vi "Periodic Tasks.vi"(8 "error in":errorcluster) -> ()   [LabVIEW 2020]
doc: "This VI runs in parallel to other tasks. It can contain as many user-defined periodic loops as you need. These can carry out PID or other sorts of timed response."
uses:
  <vilib>/Rock Robotics/WPI/ThirdParty/JAS_Junk/TrajLib/TypeDef/POSE2D.ctl
  <vilib>/Rock Robotics/WPI/ThirdParty/JAS_Junk/TrajLib/TypeDef/TRANSLATION2D.ctl
  <vilib>/Rock Robotics/WPI/ThirdParty/JAS_Junk/TrajLib/TypeDef/ROTATION2D.ctl
  <vilib>/Rock Robotics/WPI/ThirdParty/JAS_Junk/TrajLib/TypeDef/SWERVE_DRIVE_ODOMETRY.ctl
  <vilib>/Rock Robotics/WPI/ThirdParty/JAS_Junk/TrajLib/TypeDef/SWERVE_DRIVE_MODULE_POSITION.ctl
  <vilib>/Rock Robotics/WPI/ThirdParty/Phoenix-LabVIEW/Motor Controller/Controls/CTRE_Phoenix_MotorControl_ControlMode.ctl
  Robot Global Data.vi
  <vilib>/Rock Robotics/WPI/ThirdParty/Phoenix-LabVIEW/CANCoder/Get/CTRE_Phoenix_CANcoder_GetSensorData.vi
  <vilib>/Rock Robotics/WPI/ThirdParty/Phoenix-LabVIEW/Pigeon IMU/CTRE_PigeonIMU_GetAccumGyro.vi
  <vilib>/Rock Robotics/WPI/ThirdParty/Phoenix-LabVIEW/Motor Controller/Get/CTRE_Phoenix_MotorController_IntegratedSensorData_TalonFX.vi
  <vilib>/Rock Robotics/WPI/ThirdParty/JAS_Junk/TrajLib/Trajectory_Library.lvlib
panel:
  out "out SWERVE_DRIVE_ODOMETRY":T1={"POSE"={"TRANSLATION"={"X"=0.0, "Y"=0.0}, "ROTATION"={"VALUE"=0.0, "COS"=1.0, "SIN"=0.0}}, "GyroOffset"={"VALUE"=0.0, "COS"=1.0, "SIN"=0.0}, "PreviousAngle"={"VALUE"=0.0, "COS"=1.0, "SIN"=0.0}, "PrevModulePositions"=[], "NumModules"=0} {"PrevModulePositions"."Angle"."SIN" format="%13.4f"; "PrevModulePositions"."Angle"."COS" format="%13.4f"; "PrevModulePositions"."Angle"."VALUE" format="%13.4f"; "PreviousAngle"."SIN" format="%13.4f"; "PreviousAngle"."COS" format="%13.4f"; "PreviousAngle"."VALUE" format="%13.4f"; "GyroOffset"."SIN" format="%13.4f"; "GyroOffset"."COS" format="%13.4f"; "GyroOffset"."VALUE" format="%13.4f"; "POSE"."ROTATION"."SIN" format="%13.4f"; "POSE"."ROTATION"."COS" format="%13.4f"; "POSE"."ROTATION"."VALUE" format="%13.4f"; "POSE"."TRANSLATION"."Y" format="%14.3f"; "POSE"."TRANSLATION"."X" format="%14.3f"}
  out "robot POSE":T2={"TRANSLATION"={"X"=0.0, "Y"=0.0}, "ROTATION"={"VALUE"=0.0, "COS"=1.0, "SIN"=0.0}} {"ROTATION"."SIN" format="%13.4f"; "ROTATION"."COS" format="%13.4f"; "ROTATION"."VALUE" format="%13.4f"; "TRANSLATION"."Y" format="%14.3f"; "TRANSLATION"."X" format="%14.3f"}
  in  "PID gains":T6={"proportional gain (Kc)"=0.008, "integral time (Ti, min)"=0.0, "derivative time (Td, min)"=0.0} {"derivative time (Td, min)" format="%.3f"; "integral time (Ti, min)" format="%.3f"; "proportional gain (Kc)" format="%.3f"}
  in  "D":dbl
  in  "F":dbl=0.05
  in  "I":dbl
  in  "P":dbl=0.03
  out "output v":dbl
  out "Velocity (Raw Sensor Units per 100 ms)":i32
  out "velocity goal":dbl
  out "Waveform Chart":cluster{dbl, "Velocity":dbl}(graph)
  # "Azimuth PID Control"
  # "Velocity PID Control"
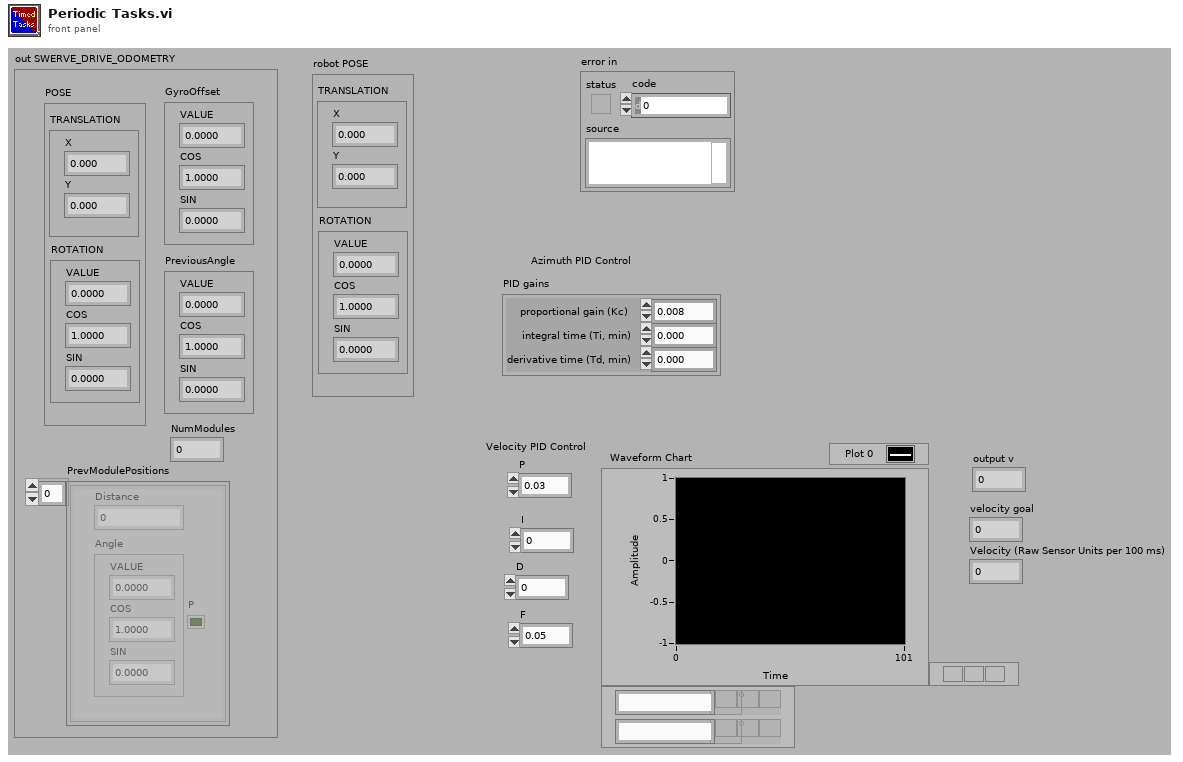
[diagram p1: front panel]
types:
  T1 = typedef "Trajectory_Library.lvlib/SWERVE_DRIVE_ODOMETRY.ctl" = cluster{"POSE":T2, "GyroOffset":T4, "PreviousAngle":T4, "PrevModulePositions":T5[], "NumModules":i32}
  T2 = typedef "Trajectory_Library.lvlib/POSE2D.ctl" = cluster{"TRANSLATION":T3, "ROTATION":T4}
  T3 = typedef "Trajectory_Library.lvlib/TRANSLATION2D.ctl" = cluster{"X":dbl, "Y":dbl}
  T4 = typedef "Trajectory_Library.lvlib/ROTATION2D.ctl" = cluster{"VALUE":dbl, "COS":dbl, "SIN":dbl}
  T5 = typedef "Trajectory_Library.lvlib/SWERVE_DRIVE_MODULE_POSITION.ctl" = cluster{"Distance":dbl, "Angle":T4, "P":bool}
  T6 = cluster{"proportional gain (Kc)":dbl, "integral time (Ti, min)":dbl, "derivative time (Td, min)":dbl}
  T7 = typedef "WPI_MotorControlDeviceRef.ctl" = cluster{"DeviceStatus":errorcluster, "Type":T8, "PWM":cluster{"PWM Channel":T9, "DeadBand":T10}, "CAN":cluster{"Device Number":u8, "SetOutput VI Ref":variant, "GetOutput VI Ref":variant, "Enable VI Ref":variant, "Disable VI Ref":variant, "Data":variant}, "Invert":bool, "DIO PWM":cluster{"PWM \"Enable\" Channel":T9, "DIOChannel":T11, "PWM Rate":dbl}}
  T8 = typedef "WPI_MotorControlType.ctl" = enum16{"PWM", "CAN", "DIO PWM"}
  T9 = typedef "FPGA_DIOPWMChannel.ctl" = enum8{"PWM 0", "PWM 1", "PWM 2", "PWM 3", "PWM 4", "PWM 5", "PWM 6", "PWM 7", "PWM 8", "PWM 9", "PWM MXP 0", "PWM MXP 1", "PWM MXP 2", "PWM MXP 3", "PWM MXP 4", "PWM MXP 5", "PWM MXP 6", "PWM MXP 7", "PWM MXP 8", "PWM MXP 9", "Invalid"}
  T10 = typedef "WPI_PWMDeadband.ctl" = cluster{"Name":string, "maxPositivePwm":i32, "minPositivePwm":i32, "centerPwm":i32, "maxNegativePwm":i32, "minNegativePwm":i32, "angularRange":u16}
  T11 = typedef "FPGA_DIOChannel.ctl" = enum8{"DIO 0", "DIO 1", "DIO 2", "DIO 3", "DIO 4", "DIO 5", "DIO 6", "DIO 7", "DIO 8", "DIO 9", "DIO MXP 0", "DIO MXP 1", "DIO MXP 2", "DIO MXP 3", "DIO MXP 4", "DIO MXP 5", "DIO MXP 6", "DIO MXP 7", "DIO MXP 8", "DIO MXP 9", "DIO MXP 10", "DIO MXP 11", "DIO MXP 12", "DIO MXP 13", "DIO MXP 14", "DIO MXP 15", "SPI Port CS1", "SPI Port CS2", "SPI Port CS3", "SPI Port MISO", "SPI Port MOSI", "Invalid"}
  T12 = typedef "CTRE_Phoenix_CANcoder_DeviceRef.ctl" = cluster{"DeviceStatus":errorcluster, "Device Number":u8, "Handle":u64, "UsageFrame":u32, "Library Path":path}
  T13 = typedef "CTRE_PigeonIMU_DeviceRef.ctl" = cluster{"DeviceStatus":errorcluster, "Device Number":u8, "Type":T14, "Device ID":u32, "Handle":u64, "UsageFrame":u32, "Library Path":path}
  T14 = typedef "CTRE_PigeonIMU_ConnectionType.ctl" = u32
  T15 = typedef "CTRE_Phoenix_MotorControl_ControlMode.ctl" = u16
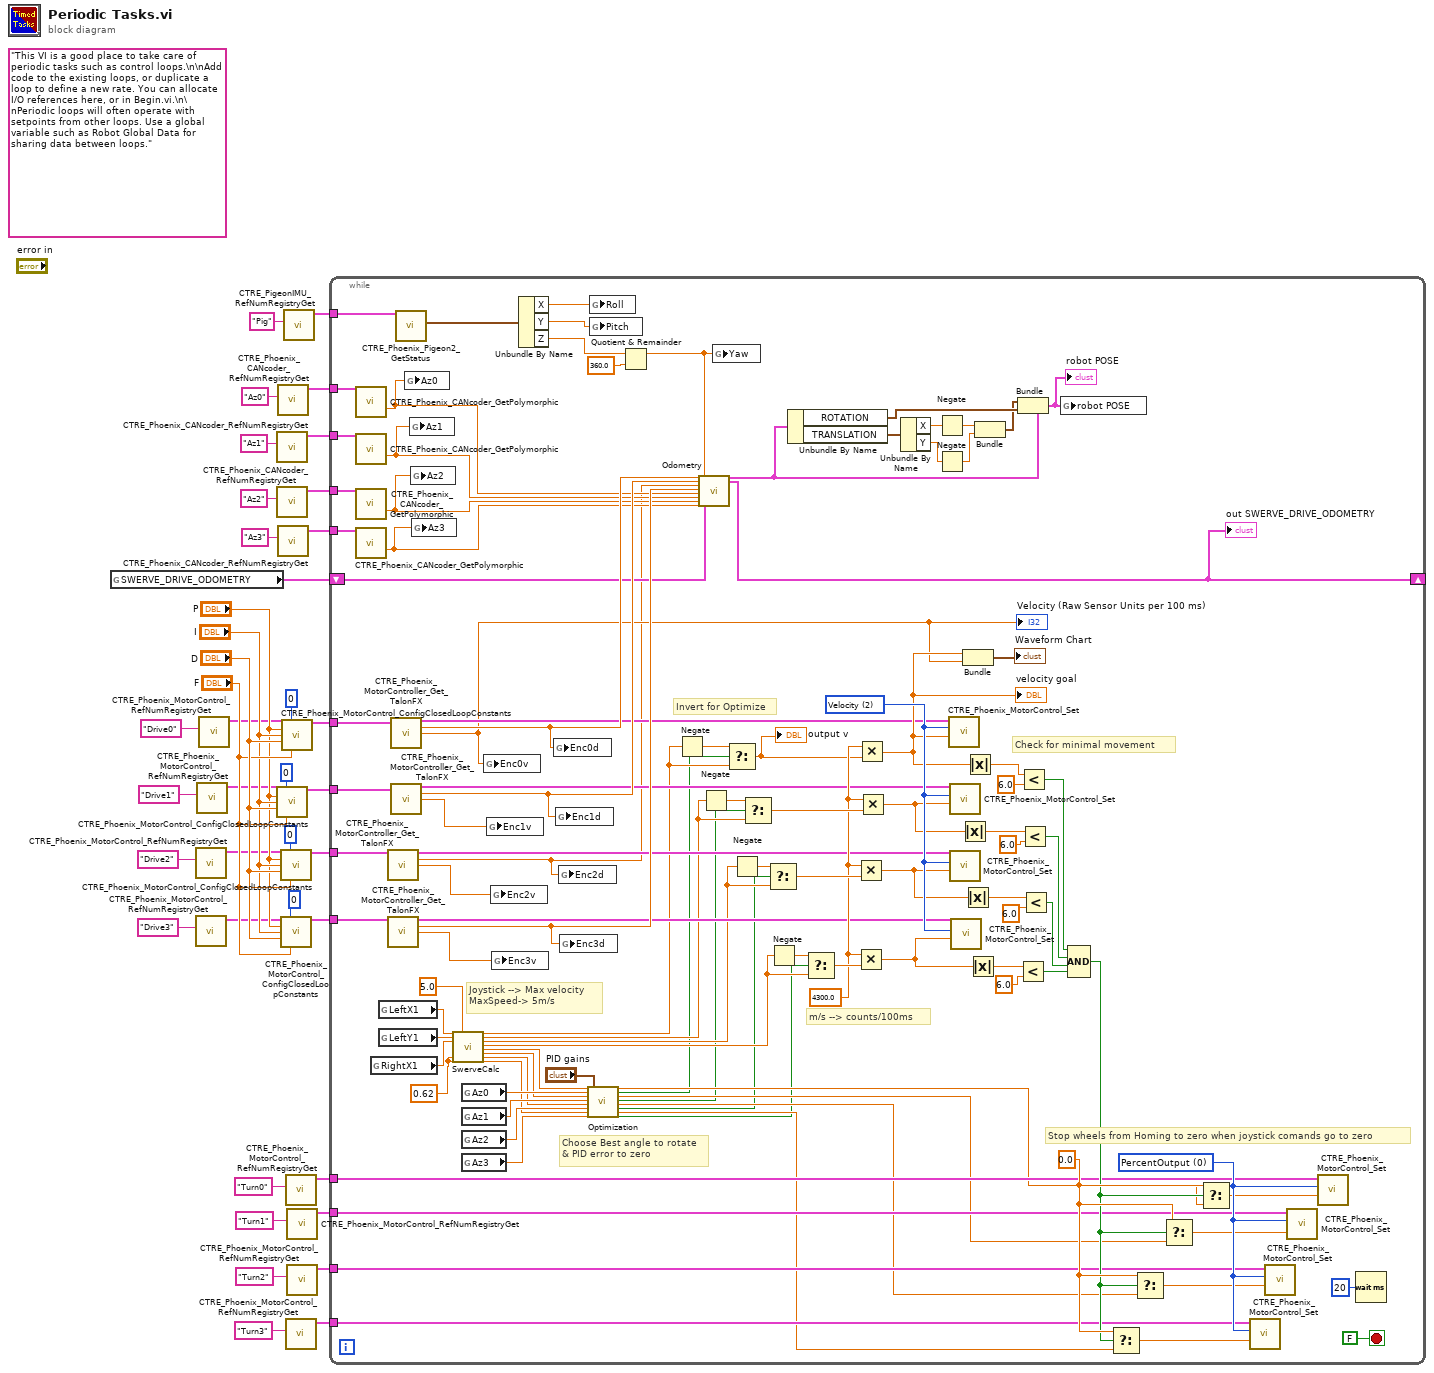
[diagram p0: block diagram]
diagram:
  (unwired) "This VI is a good place to take care of periodic tasks such as control loops.\n\nAdd code to the existing loops, or duplicate a loop to define a new rate. You can allocate I/O references here, or in Begin.vi.\n\nPeriodic loops will often operate with setpoints from other loops. Use a global variable such as Robot Global Data for sharing data between loops."
  n1 = global read "Robot Global Data.vi" "SWERVE_DRIVE_ODOMETRY"() -> (w1:T1)
  n2 = call <vilib>:"CTRE_Phoenix_MotorControl_RefNumRegistryGet.vi"("refnum name"="Drive2") -> ("PhoenixMotorControlDevRef"=w22:T7)  [unwired: 9 in, 1 out]
  n3 = call <vilib>:"CTRE_Phoenix_MotorControl_RefNumRegistryGet.vi"("refnum name"="Drive3") -> ("PhoenixMotorControlDevRef"=w24:T7)  [unwired: 9 in, 1 out]
  n4 = call <vilib>:"CTRE_Phoenix_MotorControl_RefNumRegistryGet.vi"("refnum name"="Drive1") -> ("PhoenixMotorControlDevRef"=w20:T7)  [unwired: 9 in, 1 out]
  n5 = call <vilib>:"CTRE_Phoenix_MotorControl_RefNumRegistryGet.vi"("refnum name"="Drive0") -> ("PhoenixMotorControlDevRef"=w26:T7)  [unwired: 9 in, 1 out]
  n6 = call <vilib>:"CTRE_Phoenix_CANcoder_RefNumRegistryGet.vi"("refnum name"="Az1") -> ("CTRE_CANcoder_DeviceRef"=w4:T12)  [unwired: 9 in, 1 out]
  n7 = call <vilib>:"CTRE_Phoenix_CANcoder_RefNumRegistryGet.vi"("refnum name"="Az2") -> ("CTRE_CANcoder_DeviceRef"=w3:T12)  [unwired: 9 in, 1 out]
  n8 = call <vilib>:"CTRE_Phoenix_MotorControl_ConfigClosedLoopConstants.vi"("PhoenixMotorControlDevRef"=w20, "slotIdx"=0, "P"="P", "I"="I", "D"="D", "F"="F") -> ("PhoenixMotorControlDevRef"=w17:T7)  [unwired: 8 in, 1 out]
  n9 = call <vilib>:"CTRE_Phoenix_CANcoder_RefNumRegistryGet.vi"("refnum name"="Az0") -> ("CTRE_CANcoder_DeviceRef"=w5:T12)  [unwired: 9 in, 1 out]
  n10 = call <vilib>:"CTRE_Phoenix_CANcoder_RefNumRegistryGet.vi"("refnum name"="Az3") -> ("CTRE_CANcoder_DeviceRef"=w2:T12)  [unwired: 9 in, 1 out]
  n11 = call <vilib>:"CTRE_Phoenix_MotorControl_ConfigClosedLoopConstants.vi"("PhoenixMotorControlDevRef"=w22, "slotIdx"=0, "P"="P", "I"="I", "D"="D", "F"="F") -> ("PhoenixMotorControlDevRef"=w16:T7)  [unwired: 8 in, 1 out]
  n12 = call <vilib>:"CTRE_Phoenix_MotorControl_ConfigClosedLoopConstants.vi"("PhoenixMotorControlDevRef"=w24, "slotIdx"=0, "P"="P", "I"="I", "D"="D", "F"="F") -> ("PhoenixMotorControlDevRef"=w15:T7)  [unwired: 8 in, 1 out]
  n13 = call <vilib>:"CTRE_Phoenix_MotorControl_ConfigClosedLoopConstants.vi"("PhoenixMotorControlDevRef"=w26, "slotIdx"=0, "P"="P", "I"="I", "D"="D", "F"="F") -> ("PhoenixMotorControlDevRef"=w18:T7)  [unwired: 8 in, 1 out]
  n14 = call <vilib>:"CTRE_PigeonIMU_RefNumRegistryGet.vi"("refnum name"="Pig") -> ("PigeonIMUDevRef"=w6:T13)  [unwired: 9 in, 1 out]
  n15 = call <vilib>:"CTRE_Phoenix_MotorControl_RefNumRegistryGet.vi"("refnum name"="Turn0") -> ("PhoenixMotorControlDevRef"=w10:T7)  [unwired: 9 in, 1 out]
  n16 = call <vilib>:"CTRE_Phoenix_MotorControl_RefNumRegistryGet.vi"("refnum name"="Turn3") -> ("PhoenixMotorControlDevRef"=w7:T7)  [unwired: 9 in, 1 out]
  n17 = call <vilib>:"CTRE_Phoenix_MotorControl_RefNumRegistryGet.vi"("refnum name"="Turn1") -> ("PhoenixMotorControlDevRef"=w9:T7)  [unwired: 9 in, 1 out]
  n18 = call <vilib>:"CTRE_Phoenix_MotorControl_RefNumRegistryGet.vi"("refnum name"="Turn2") -> ("PhoenixMotorControlDevRef"=w8:T7)  [unwired: 9 in, 1 out]
  n19 = while {
    tunnel: w18 -> [w114]
    tunnel: w17 -> [w113]
    tunnel: w16 -> [w112]
    tunnel: w15 -> [w111]
    tunnel: w10 -> [w98]
    tunnel: w9 -> [w97]
    tunnel: w8 -> [w96]
    tunnel: w7 -> [w95]
    tunnel: w6 -> [w56]
    tunnel: w5 -> [w55]
    tunnel: w4 -> [w54]
    tunnel: w3 -> [w53]
    tunnel: w2 -> [w52]
    shift-right: [w50] -> _
    shift-left: w1 -> [w51]
    stop <- FALSE stop-if-true
    w103 = 0.0 ("t")
    w68 = 0.62 ("Width")
    w105 = T15 0 items=["PercentOutput"=0, "Position"=1, "Velocity"=2, "Current"=3, "Follower"=5, "MotionProfile"=6, "MotionMagic"=7, "MotionProfileArc"=10, "Disabled"=15] ("Control Mode")
    w121 = 4300.0 ("y")
    w140 = T15 2 items=["PercentOutput"=0, "Position"=1, "Velocity"=2, "Current"=3, "Follower"=5, "MotionProfile"=6, "MotionMagic"=7, "MotionProfileArc"=10, "Disabled"=15] ("Control Mode")
    # "Choose Best angle to rotate\n& PID error to zero"
    # "Joystick --> Max velocity\nMaxSpeed-> 5m/s"
    # "Stop wheels from Homing to zero when joystick comands go to zero"
    # "Invert for Optimize"
    # "m/s --> counts/100ms"
    # "Check for minimal movement"
    n20 = call-poly <vilib>:"CTRE_Phoenix_CANcoder_GetPolymorphic.vi"("CTRE_CANcoder_DeviceRef"=w55) -> ("Absolute Position"=w60:dbl)  [unwired: 10 in, 4 out]
    n21 = call-poly <vilib>:"CTRE_Phoenix_CANcoder_GetPolymorphic.vi"("CTRE_CANcoder_DeviceRef"=w54) -> ("Absolute Position"=w59:dbl)  [unwired: 10 in, 4 out]
    n22 = call-poly <vilib>:"CTRE_Phoenix_CANcoder_GetPolymorphic.vi"("CTRE_CANcoder_DeviceRef"=w53) -> ("Absolute Position"=w58:dbl)  [unwired: 10 in, 4 out]
    n23 = call-poly <vilib>:"CTRE_Phoenix_CANcoder_GetPolymorphic.vi"("CTRE_CANcoder_DeviceRef"=w52) -> ("Absolute Position"=w57:dbl)  [unwired: 10 in, 4 out]
    n24 = global read "Robot Global Data.vi" "RightX1"() -> (w91:dbl)
    n25 = global read "Robot Global Data.vi" "LeftX1"() -> (w93:dbl)
    n26 = global read "Robot Global Data.vi" "LeftY1"() -> (w92:dbl)
    n27 = call-poly <vilib>:"CTRE_Phoenix_MotorController_Get_TalonFX.vi"("PhoenixMotorControlDevRef"=w112) -> ("PhoenixMotorControlDevRef"=w116:T7, "Position"=w49:dbl, "Velocity"=w109:dbl)  [unwired: 10 in, 2 out]
    n28 = call-poly <vilib>:"CTRE_Phoenix_MotorController_Get_TalonFX.vi"("PhoenixMotorControlDevRef"=w111) -> ("PhoenixMotorControlDevRef"=w115:T7, "Position"=w122:dbl, "Velocity"=w108:dbl)  [unwired: 10 in, 2 out]
    n29 = call-poly <vilib>:"CTRE_Phoenix_MotorController_Get_TalonFX.vi"("PhoenixMotorControlDevRef"=w114) -> ("PhoenixMotorControlDevRef"=w118:T7, "Position"=w120:dbl, "Velocity"=w110:dbl)  [unwired: 10 in, 2 out]
    "Velocity (Raw Sensor Units per 100 ms)" <- w110
    n30 = call-poly <vilib>:"CTRE_Phoenix_MotorController_Get_TalonFX.vi"("PhoenixMotorControlDevRef"=w113) -> ("PhoenixMotorControlDevRef"=w117:T7, "Position"=w123:dbl, "Velocity"=w107:dbl)  [unwired: 10 in, 2 out]
    n31 = call-poly <vilib>:"CTRE_Phoenix_Pigeon2_GetStatus.vi"("PigeonIMUDevRef"=w56) -> ("AccumGyro"=w66:cluster{"X":dbl, "Y":dbl, "Z":dbl})  [unwired: 8 in, 2 out]
    n32 = global write "Robot Global Data.vi" "Az0"(w60) -> ()
    n33 = global write "Robot Global Data.vi" "Az1"(w59) -> ()
    n34 = global write "Robot Global Data.vi" "Az2"(w58) -> ()
    n35 = global write "Robot Global Data.vi" "Az3"(w57) -> ()
    n36 = call "SwerveCalc.vi"("Jx"=w93, "Jy"=w92, "Jr"=w91, "Length"=w68, "Width"=w68, "MaxV"=5.0) -> ("V0"=w81:dbl, "V1"=w80:dbl, "V2"=w79:dbl, "V3"=w78:dbl, "A0"=w89:dbl, "A1"=w87:dbl, "A2"=w85:dbl, "A3"=w83:dbl)  [unwired: 14 in]
    n37 = global read "Robot Global Data.vi" "Az0"() -> (w88:dbl)
    n38 = global read "Robot Global Data.vi" "Az1"() -> (w86:dbl)
    n39 = global read "Robot Global Data.vi" "Az2"() -> (w84:dbl)
    n40 = global read "Robot Global Data.vi" "Az3"() -> (w82:dbl)
    n41 = global write "Robot Global Data.vi" "Enc0v"(w110) -> ()
    n42 = global write "Robot Global Data.vi" "Enc1v"(w107) -> ()
    n43 = global write "Robot Global Data.vi" "Enc2v"(w109) -> ()
    n44 = global write "Robot Global Data.vi" "Enc3v"(w108) -> ()
    n45 = Unbundle By Name(w66) -> ("X"=w61:dbl, "Y"=w62:dbl, "Z"=w64:dbl)
    n46 = global write "Robot Global Data.vi" "Enc0d"(w120) -> ()
    n47 = global write "Robot Global Data.vi" "Enc1d"(w123) -> ()
    n48 = global write "Robot Global Data.vi" "Enc2d"(w49) -> ()
    n49 = global write "Robot Global Data.vi" "Enc3d"(w122) -> ()
    n50 = call "Optimization.vi"("GoalAngle0"=w89, "Az0"=w88, "GoalAngle1"=w87, "Az1"=w86, "GoalAngle2"=w85, "Az2"=w84, "GoalAngle3"=w83, "Az3"=w82, "PID gains"="PID gains") -> ("A0"=w77:dbl, "Flip0"=w73:bool, "A1"=w76:dbl, "Flip1"=w72:bool, "A2"=w75:dbl, "Flip2"=w71:bool, "A3"=w74:dbl, "Flip3"=w70:bool)  [unwired: 11 in]
    n51 = global write "Robot Global Data.vi" "Roll"(w61) -> ()
    n52 = global write "Robot Global Data.vi" "Pitch"(w62) -> ()
    n53 = Quotient & Remainder(x=w64, y=360.0) -> (x-y*floor(x/y)=w63:dbl)  [unwired: 1 out]
    n54 = Negate(x=w81) -> (-x=w145:dbl)
    n55 = call "Odometry.vi"("Enc0"=w120, "Enc1"=w123, "Enc2"=w49, "Enc3"=w122, "Az0"=w60, "Az1"=w59, "Az2"=w58, "Az3"=w57, "Heading"=w63, "in SWERVE_DRIVE_ODOMETRY"=w51) -> ("robot POSE"=w43:T2, "out SWERVE_DRIVE_ODOMETRY"=w50:T1)  [unwired: 16 in]
    "out SWERVE_DRIVE_ODOMETRY" <- w50
    n56 = Negate(x=w80) -> (-x=w146:dbl)
    n57 = global write "Robot Global Data.vi" "Yaw"(w63) -> ()
    n58 = Select(t=w145, s=w73, f=w81) -> (s? t:f=w119:dbl)
    "output v" <- w119
    n59 = Negate(x=w79) -> (-x=w144:dbl)
    n60 = Select(t=w146, s=w72, f=w80) -> (s? t:f=w147:dbl)
    n61 = Select(t=w144, s=w71, f=w79) -> (s? t:f=w143:dbl)
    n62 = Negate(x=w78) -> (-x=w142:dbl)
    n63 = Unbundle By Name(w43) -> ("ROTATION"=w42:T4, "TRANSLATION"=w48:T3)
    n64 = Select(t=w142, s=w70, f=w78) -> (s? t:f=w141:dbl)
    n65 = Multiply(x=w121, y=w143) -> (x*y=w131:dbl)
    n66 = Multiply(x=w121, y=w141) -> (x*y=w130:dbl)
    n67 = Multiply(x=w121, y=w119) -> (x*y=w139:dbl)
    "velocity goal" <- w139
    n68 = Multiply(x=w121, y=w147) -> (x*y=w132:dbl)
    n69 = Unbundle By Name(w48) -> ("X"=w47:dbl, "Y"=w46:dbl)
    n70 = Negate(x=w47) -> (-x=w44:dbl)
    n71 = Negate(x=w46) -> (-x=w45:dbl)
    n72 = call <vilib>:"CTRE_Phoenix_MotorControl_Set.vi"("Output"=w139, "Control Mode"=w140, "PhoenixMotorControlDevRef"=w118) -> ()  [unwired: 7 in, 2 out]
    n73 = call <vilib>:"CTRE_Phoenix_MotorControl_Set.vi"("Output"=w132, "Control Mode"=w140, "PhoenixMotorControlDevRef"=w117) -> ()  [unwired: 7 in, 2 out]
    n74 = call <vilib>:"CTRE_Phoenix_MotorControl_Set.vi"("Output"=w131, "Control Mode"=w140, "PhoenixMotorControlDevRef"=w116) -> ()  [unwired: 7 in, 2 out]
    n75 = call <vilib>:"CTRE_Phoenix_MotorControl_Set.vi"("Output"=w130, "Control Mode"=w140, "PhoenixMotorControlDevRef"=w115) -> ()  [unwired: 7 in, 2 out]
    n76 = Absolute Value(x=w132) -> (abs(x)=w125:dbl)
    n77 = Bundle(w139, "Velocity"=w110) -> (→"Waveform Chart":cluster{dbl, "Velocity":dbl})  [unwired: 1 in]
    n78 = Absolute Value(x=w131) -> (abs(x)=w126:dbl)
    n79 = Absolute Value(x=w139) -> (abs(x)=w124:dbl)
    n80 = Absolute Value(x=w130) -> (abs(x)=w127:dbl)
    n81 = Bundle(w44, w45) -> (w41:cluster{dbl, dbl})  [unwired: 1 in]
    n82 = Bundle(cluster=w43, "TRANSLATION"=w41, "ROTATION"=w42) -> (w40:T2)
    "robot POSE" <- w40
    n83 = Less?(x=w127, y=6.0) -> (x < y?=w134:bool)
    n84 = Less?(x=w124, y=6.0) -> (x < y?=w137:bool)
    n85 = Less?(x=w125, y=6.0) -> (x < y?=w136:bool)
    n86 = Less?(x=w126, y=6.0) -> (x < y?=w135:bool)
    n87 = global write "Robot Global Data.vi" "robot POSE"(w40) -> ()
    n88 = Compound Arithmetic op=AND(w137, w136, w135, w134) -> (w99:bool)
    n89 = Select(t=w103, s=w99, f=w74) -> (s? t:f=w100:dbl)
    n90 = Select(t=w103, s=w99, f=w75) -> (s? t:f=w101:dbl)
    n91 = Select(t=w103, s=w99, f=w76) -> (s? t:f=w102:dbl)
    n92 = Select(t=w103, s=w99, f=w77) -> (s? t:f=w104:dbl)
    n93 = call <vilib>:"CTRE_Phoenix_MotorControl_Set.vi"("Output"=w100, "Control Mode"=w105, "PhoenixMotorControlDevRef"=w95) -> ()  [unwired: 7 in, 2 out]
    n94 = call <vilib>:"CTRE_Phoenix_MotorControl_Set.vi"("Output"=w101, "Control Mode"=w105, "PhoenixMotorControlDevRef"=w96) -> ()  [unwired: 7 in, 2 out]
    n95 = call <vilib>:"CTRE_Phoenix_MotorControl_Set.vi"("Output"=w102, "Control Mode"=w105, "PhoenixMotorControlDevRef"=w97) -> ()  [unwired: 7 in, 2 out]
    n96 = call <vilib>:"CTRE_Phoenix_MotorControl_Set.vi"("Output"=w104, "Control Mode"=w105, "PhoenixMotorControlDevRef"=w98) -> ()  [unwired: 7 in, 2 out]
    n97 = Wait (ms)(milliseconds to wait=u32 20) -> ()  [unwired: 1 out]
  }
